vi "Implement Publication Policy.vi"(5 "Last Published Value":variant, 7 "Last Published Time":timestamp, 9 "New Value Time":timestamp, 10 "New Value":variant, 11 "MergeErrorsPublication":refnum<class "MergeErrorsPublication.lvclass">) -> (0 "error out (Reject Publication)":errorcluster, 2 "Value to Publish":variant)   [LabVIEW 2019, in "PublicationPolicy.lvlib" / "MergeErrorsPublication.lvclass"]
doc: "This method decides whether or not to send or otherwise handle the new data value. The policy is set and maintained by the subscriber. The Topic Actor knows no policy details, it just passes the new value in. If there is a failure inside this method, the Topic Actor must assume the listener is no longer valid (dead/unrecoverable) and should delete it from the Subscriber list.\n\n<License>\nCopyright © 2017 Composed Systems, LLC | All rights reserved\nwww.composed.io\n\nAuthor: Ethan Stern <ethan.stern@composed.io>\n\nThis software is provided \"AS IS\" WITHOUT WARRANTIES, either express or implied, AND IS FOR EDUCATIONAL PURPOSES ONLY.\n</License>"
uses:
  <vilib>/gpm_packages/@cs/mva-core/Source/PublicationPolicy/MergeErrorsPublication/MergeErrorsPublication.lvclass
  <vilib>/ErrorRing/Error Ring.xnode
  <vilib>/Utility/Data Type/NI_Data Type.lvlib
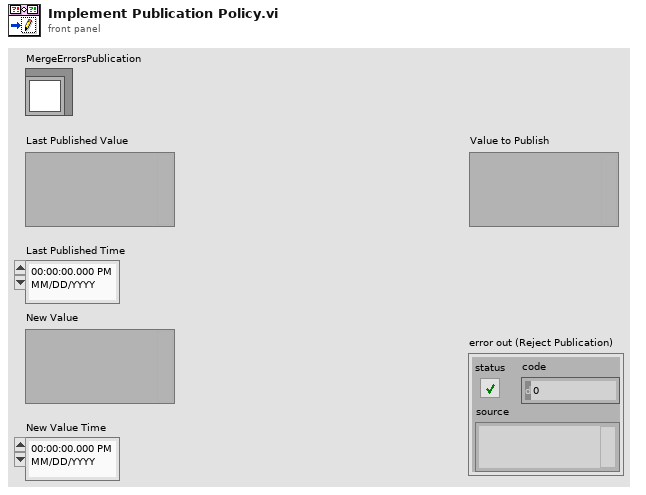
[diagram p1: front panel]
types:
  T1 = typedef "NI_Data Type.lvlib/Data Type.ctl" = enum8{"Invalid Type", "Void", "I8", "I16", "I32", "I64", "U8", "U16", "U32", "U64", "Single Float", "Double Float", "Extended Float", "Single Complex", "Double Complex", "Extended Complex", "Enum U8", "Enum U16", "Enum U32", "Enum U64", "Single Float With Unit", "Double Float With Unit", "Extended Float With Unit", "Single Complex with Unit", "Double Complex with Unit", "Extended Complex with Unit", "Boolean", "String", "Path", "Picture", "Tag", "Array", "Cluster", "Variant", "LV Variant", "Waveform", "Timestamp", "Digital Waveform", "Digital Data", "ExpressData", "Refnum", "External Data", "VI", "Poly VI", "LabVIEW Class Instance", "Fixed Point", "Set Collection", "Map Collection"}
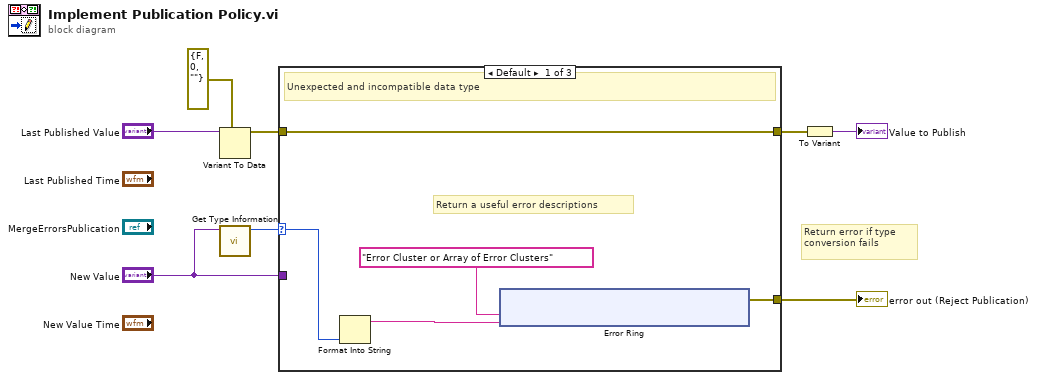
[diagram p0: block diagram]
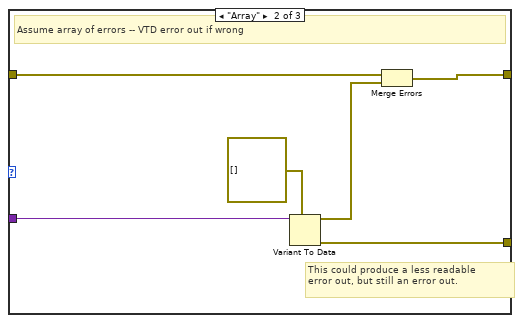
[diagram p2: hidden frame]
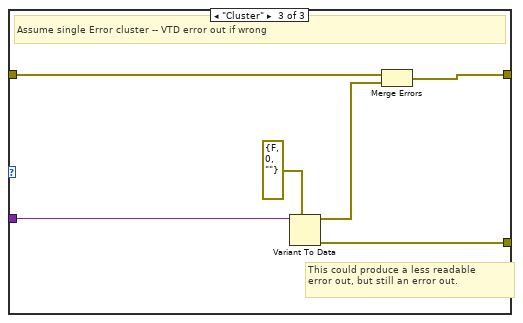
[diagram p3: hidden frame]
diagram:
  # "Return error if type\nconversion fails"
  n1 = Variant To Data(type=errorcluster {"status"=FALSE, "code"=0, "source"=""} ("error constant"), Variant="Last Published Value") -> (data=w7:errorcluster)  [unwired: 1 in, 1 out]
  n2 = call <vilib>:"Get Type Information.vi"("variant"="New Value") -> ("type"=w5:T1)  [unwired: 6 in, 4 out]
  n3 = case shown="Default" w5 {
    selector: w5 -> [w11 _ _]
    tunnel: w7 -> [w13 w25 w31]
    tunnel: "New Value" -> [_ w24 w30]
    tunnel: [w13 w21 w27] -> w2
    tunnel: [w12 w20 w26] -> w4
    frame Default {
      # "Return a useful error descriptions"
      # "Unexpected and incompatible data type"
      n4 = Format Into String(w11) -> (resulting string=w10:string)  [unwired: 3 in, 1 out]
      n5 = xnode "Error Ring"("parameter 0"="Error Cluster or Array of Error Clusters", "parameter 1"=w10) -> ("error out"=w12:errorcluster)
    }
    frame "Array" {
      # "This could produce a less readable\nerror out, but still an error out."
      # "Assume array of errors -- VTD error out if wrong"
      n6 = Variant To Data(type=errorcluster[] [] ("error constant"), Variant=w24) -> (data=w22:errorcluster[], error out=w20:errorcluster)  [unwired: 1 in]
      n7 = Merge Errors(w25, w22) -> (w21:errorcluster)
    }
    frame "Cluster" {
      # "This could produce a less readable\nerror out, but still an error out."
      # "Assume single Error cluster -- VTD error out if wrong"
      n8 = Variant To Data(type=errorcluster {"status"=FALSE, "code"=0, "source"=""} ("error constant"), Variant=w30) -> (data=w28:errorcluster, error out=w26:errorcluster)  [unwired: 1 in]
      n9 = Merge Errors(w31, w28) -> (w27:errorcluster)
    }
  }
  "error out (Reject Publication)" <- w4
  n10 = To Variant(anything=w2) -> (Variant=→"Value to Publish":variant)
